vi "Element Events.vi"(8 "error in (no error)":errorcluster, 11 "BooleanControl in":refnum<class "BooleanControl.lvclass">) -> (0 "error out":errorcluster, 2 "Element Events":refnum<class "Control Event Registrations.lvclass">, 3 "BooleanControl out":refnum<class "BooleanControl.lvclass">)   [LabVIEW 2020, in "VolatusGUIElements.lvlib" / "BooleanControl.lvclass"]
uses:
  BooleanControl.lvclass
  C:/dev/lv20CE/relink/lv-volatus/VolatusGUI/GUI Element/GUI Element.lvclass
  C:/dev/lv20CE/relink/lv-volatus/VolatusGUI/OnValueChangeHandler/OnValueChangeHandler.lvclass
  VolatusGUI/Control Event Registrations/Control Event Registrations.lvclass
  VolatusGUI/GUI Element/GUI Element.lvclass/GUI Element.ctl
  BooleanControl.lvclass/BooleanControl.ctl
  VolatusGUI/GUI Element/GUI Element.lvclass
  C:/dev/lv20CE/relink/lv-volatus/VolatusGUIElements/BooleanControl/BooleanControl.lvclass
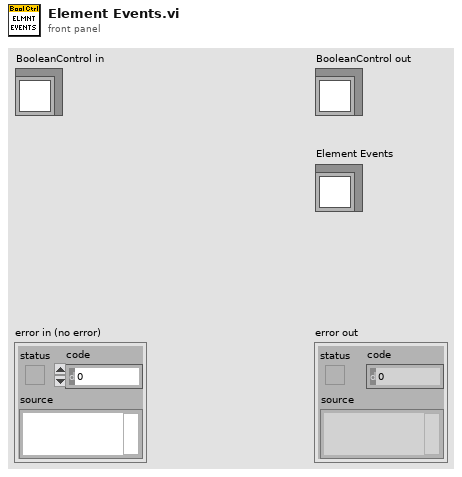
[diagram p1: front panel]
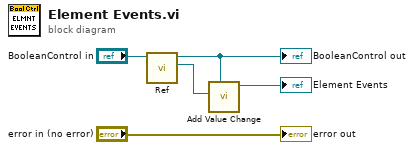
[diagram p0: block diagram]
diagram:
  n1 = call "Ref.vi"("GUI Element in"="BooleanControl in") -> ("Ref"=w1:refnum<vi>, "GUI Element out"=w2:refnum<class "BooleanControl.lvclass">)  [unwired: 9 in]
  "BooleanControl out" <- w2
  n2 = call "Add Value Change.vi"("Control"=w2, "CtlRef"=w1) -> ("Control Event Registrations out"=→"Element Events":refnum<class "Control Event Registrations.lvclass">)  [unwired: 8 in, 1 out]
  "error out" <- "error in (no error)"
